vi "DAQNavi Read (Counter 1D Frequency 1Chan NSamp).vi"(8 "error in (no error)":errorcluster, 9 "number of samples per channel to read":u32=10, 10 "timeout":dbl=10.0, 11 "task in":i32) -> (0 "error out":errorcluster, 2 "data":dbl[](array[numeric]), 3 "task out":i32)   [LabVIEW 2020]
uses:
  DAQNavi_LV.dll
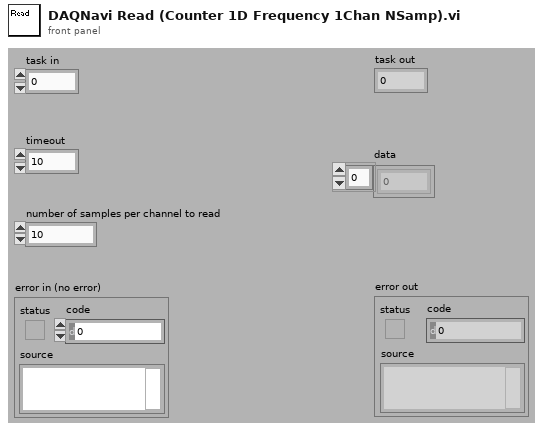
[diagram p1: front panel]
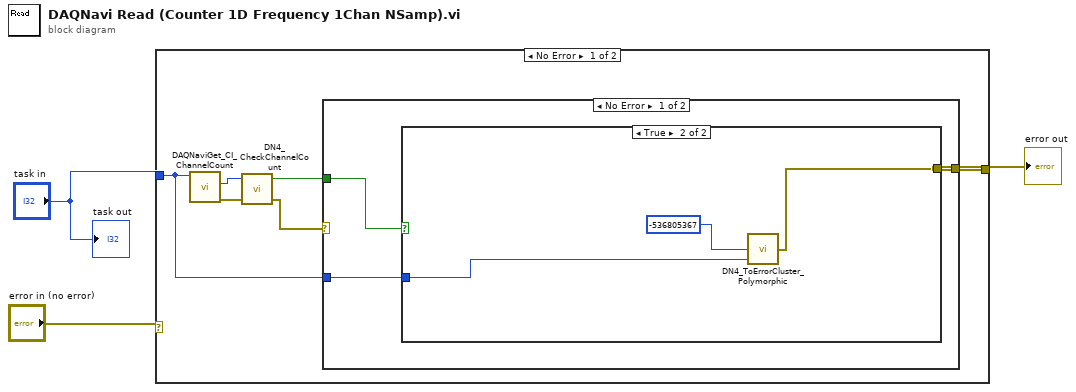
[diagram p0: block diagram]
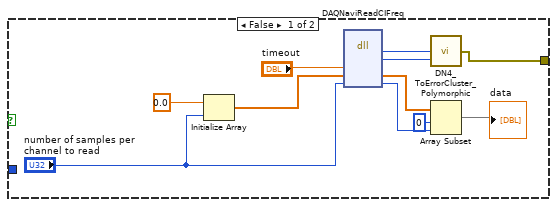
[diagram p2: hidden frame]
diagram:
  n1 = case shown="No Error" "error in (no error)" {
    selector: "error in (no error)" -> [_ w28]
    tunnel: "task in" -> [w4 _]
    tunnel: [w9 w28] -> w1
    frame No Error {
      n2 = call "DAQNaviGet_CI_ChannelCount.vi"("task in"=w4) -> ("error out"=w8:errorcluster, "channel count"=w7:i32)  [unwired: 1 in, 8 out]
      n3 = call "DN4_CheckChannelCount.vi"("error out"=w8, "channel count"=w7) -> ("error IO"=w6:errorcluster, "greater than 1?"=w5:bool)  [unwired: 2 out]
      n4 = case shown="No Error" w6 {
        selector: w6 -> [_ w27]
        tunnel: [w12 w27] -> w9
        tunnel: w5 -> [w11 _]
        tunnel: w4 -> [w10 _]
        frame No Error {
          n5 = case shown="True" w11 {
            tunnel: [w13 w24] -> w12
            tunnel: w10 -> [_ w25]
            frame False {
              n6 = Initialize Array(0.0 ("element"), "number of samples per channel to read") -> (w15:dbl[])
              n7 = dll-call lib="DAQNavi_LV.dll" fn="DAQNaviReadCIFreq"("timeout"="timeout", "freq"=w15, "samples"="number of samples per channel to read") -> ("return type"=w23:i32, "taskID"=w14:i32, "freq"=w21:dbl[], "samples"=w19:u32)  [unwired: 4 in, 3 out]
              n8 = call "DN4_ToErrorCluster_Polymorphic.vi"("task id"=w14, "error code"=w23) -> ("error out"=w13:errorcluster)  [unwired: 3 out]
              n9 = Array Subset(array=w21, index=0, length=w19) -> (→"data":dbl[])
            }
            frame True {
              n10 = call "DN4_ToErrorCluster_Polymorphic.vi"("task id"=w25, "error code"=-536805367 ("error code (0)")) -> ("error out"=w24:errorcluster)  [unwired: 3 out]
            }
          }
        }
        frame Error {
        }
      }
    }
    frame Error {
    }
  }
  "error out" <- w1
  "task out" <- "task in"
